vi "Control and indicators refs.vi"() -> ()   [LabVIEW 2021]
uses:
  Typedefs/Control and indicators refs.ctl
panel:
  in  "Controls":T1
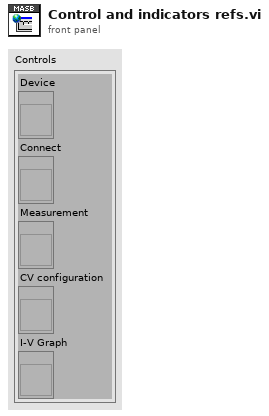
[diagram p1: front panel]
types:
  T1 = typedef "Control and indicators refs.ctl" = cluster{"Device":refnum<vi>, "Connect":refnum<vi>, "Measurement":refnum<vi>, "CV configuration":refnum<vi>, "I-V Graph":refnum<vi>}
diagram:
